vi "Overlay.vi"(0 "Image In":T5, 5 "Overlay Details":T4={"Measurment Name"="", "Measurment Type"="", "Image ID"="", "Result"=[], "PointForOverlays"={"Line"=[], "Angle"=[], "Circle"=[], "Points"={"Points"=[]}, "Coordinate System"={"Origin"={"X"=0.0, "Y"=0.0}, "Angle (deg)"=0.0, "Axis Reference"=0}}, "Color"=16748288, "Mouse coordinates"={"X"=0.0, "Y"=0.0}, "Inspect Overlay Coordinate"=[], "Angle of rotation"=0.0} {"Inspect Overlay Coordinate"."Y" format="%.2f"; "Inspect Overlay Coordinate"."X" format="%.2f"; "Mouse coordinates"."Y" format="%.2f"; "Mouse coordinates"."X" format="%.2f"; "PointForOverlays"."Coordinate System"."Axis Reference" items=["Direct", "Indirect"]; "PointForOverlays"."Coordinate System"."Angle (deg)" format="%.2f"; "PointForOverlays"."Coordinate System"."Origin"."Y" format="%.2f"; "PointForOverlays"."Coordinate System"."Origin"."X" format="%.2f"; "PointForOverlays"."Points"."Points"."Y" format="%.2f"; "PointForOverlays"."Points"."Points"."X" format="%.2f"; "PointForOverlays"."Circle"."Point 2"."Y" format="%.2f"; "PointForOverlays"."Circle"."Point 2"."X" format="%.2f"; "PointForOverlays"."Circle"."Point 1"."Y" format="%.2f"; "PointForOverlays"."Circle"."Point 1"."X" format="%.2f"; "PointForOverlays"."Angle"."line2Point2"."Y" format="%.2f"; "PointForOverlays"."Angle"."line2Point2"."X" format="%.2f"; "PointForOverlays"."Angle"."line2Point1"."Y" format="%.2f"; "PointForOverlays"."Angle"."line2Point1"."X" format="%.2f"; "PointForOverlays"."Angle"."line1Point2"."Y" format="%.2f"; "PointForOverlays"."Angle"."line1Point2"."X" format="%.2f"; "PointForOverlays"."Angle"."line1Point1"."Y" format="%.2f"; "PointForOverlays"."Angle"."line1Point1"."X" format="%.2f"; "PointForOverlays"."Angle"."Point 2a"."Y" format="%.2f"; "PointForOverlays"."Angle"."Point 2a"."X" format="%.2f"; "PointForOverlays"."Angle"."Point 1a"."Y" format="%.2f"; "PointForOverlays"."Angle"."Point 1a"."X" format="%.2f"; "PointForOverlays"."Angle"."vertex"."Y" format="%.2f"; "PointForOverlays"."Angle"."vertex"."X" format="%.2f"; "PointForOverlays"."Angle"."Point 2"."Y" format="%.2f"; "PointForOverlays"."Angle"."Point 2"."X" format="%.2f"; "PointForOverlays"."Angle"."Point 1"."Y" format="%.2f"; "PointForOverlays"."Angle"."Point 1"."X" format="%.2f"; "PointForOverlays"."Line"."Point 2"."Y" format="%.2f"; "PointForOverlays"."Line"."Point 2"."X" format="%.2f"; "PointForOverlays"."Line"."Point 1"."Y" format="%.2f"; "PointForOverlays"."Line"."Point 1"."X" format="%.2f"}, 7 "Testing Parameters":T1={"Stored overlay coordinates"=[], "Testing?"=TRUE}, 9 "Overlay Cluster":T3, 11 "error in":errorcluster) -> (4 "Image Out":T5, 6 "Overlay output":T2, 15 "error out":errorcluster)   [LabVIEW 2015]
uses:
  <vilib>/vision/Image Controls.llb/IMAQ Image.ctl
  Controls/overlayWithDetails.ctl
  Controls/Overlay Cluster.ctl
  Controls/Overlay output.ctl
  Controls/Testing parameters.ctl
  Controls/User inputs (line).ctl
  Controls/Calculated inputs (line).ctl
  Controls/Angle details.ctl
  Controls/Circle dia data.ctl
  Controls/DatumLine draw.ctl
  Controls/GD&T overlay.ctl
panel:
  in  "Xoffset":i32
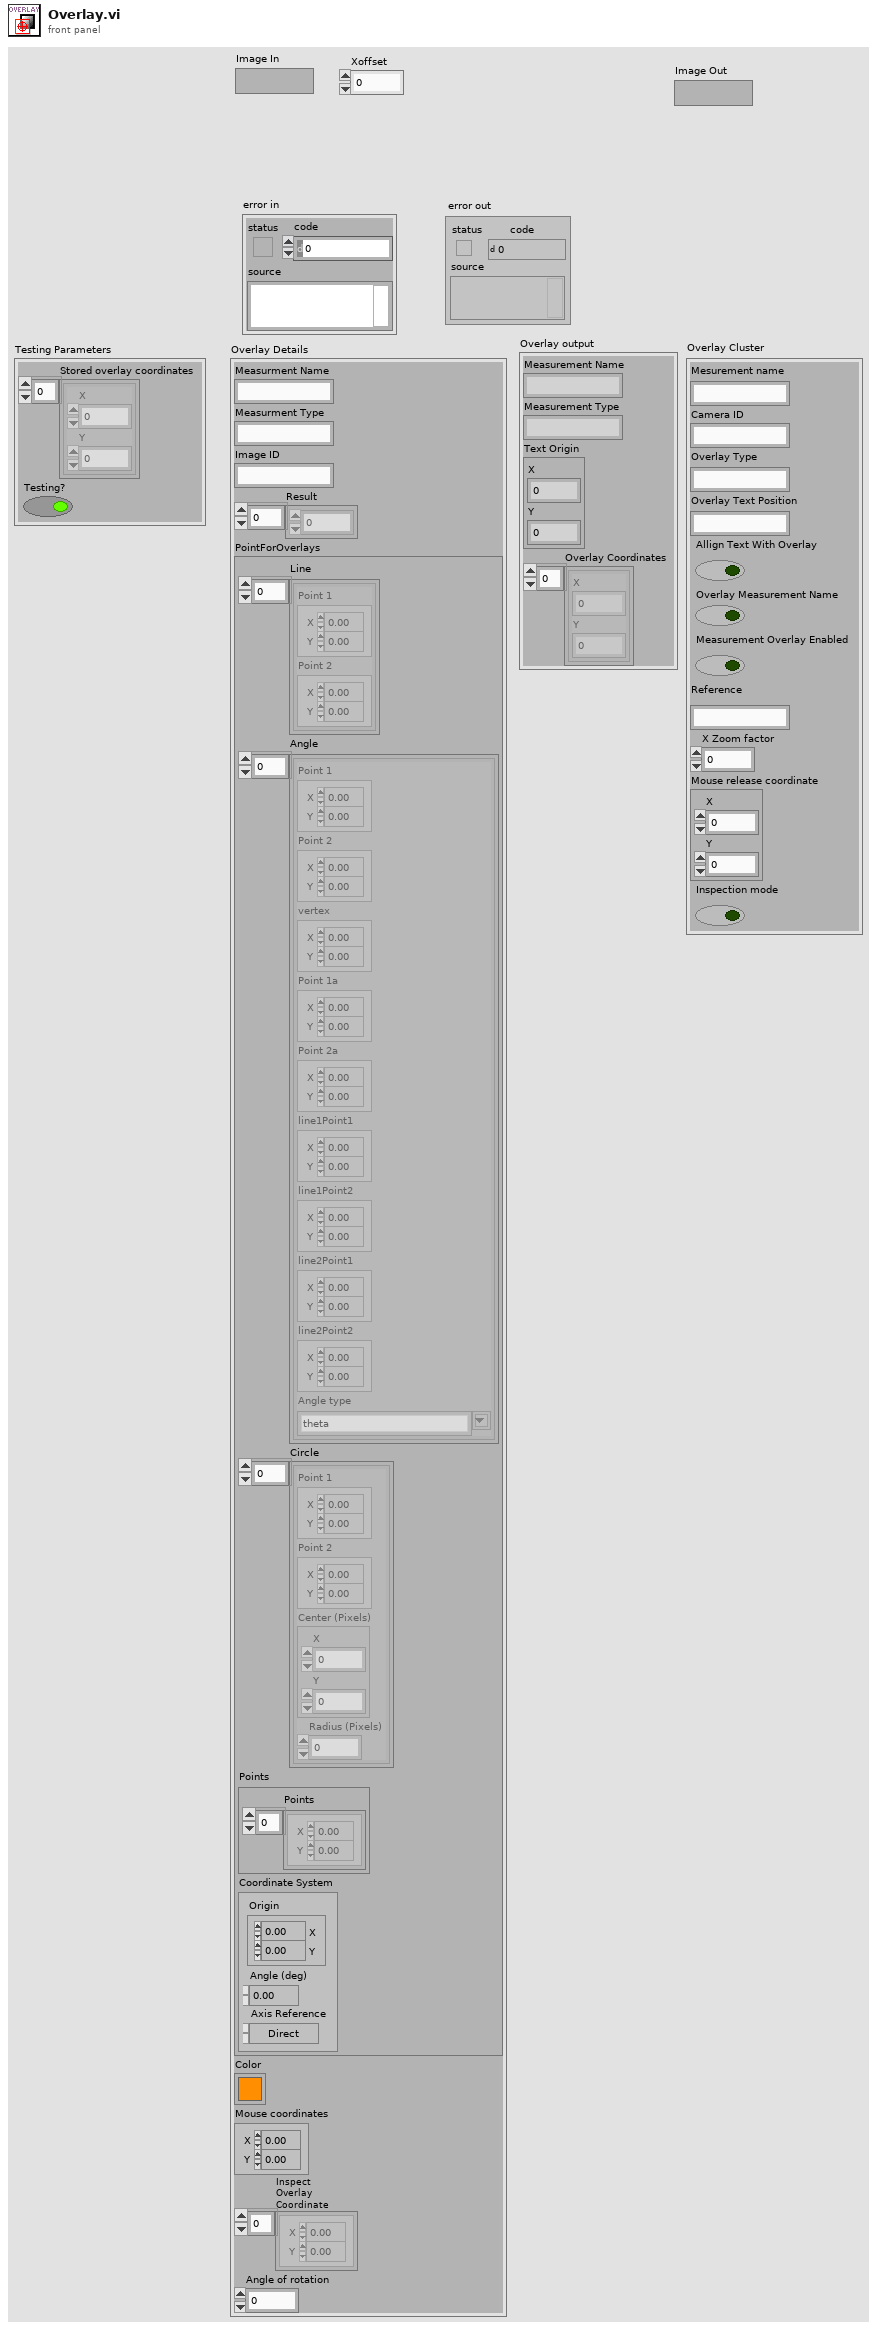
[diagram p1: front panel]
types:
  T1 = typedef "Testing parameters.ctl" = cluster{"Stored overlay coordinates":cluster{"X":sgl, "Y":sgl}[], "Testing?":bool}
  T2 = typedef "Overlay output.ctl" = cluster{"Measurement Name":string, "Measurement Type":string, "Text Origin":cluster{"X":dbl, "Y":dbl}, "Overlay Coordinates":cluster{"X":sgl, "Y":sgl}[]}
  T3 = typedef "Overlay Cluster.ctl" = cluster{"Mesurement name":string, "Camera ID":string, "Overlay Type":string, "Overlay Text Position":string, "Allign Text With Overlay":bool, "Overlay Measurement Name":bool, "Measurement Overlay Enabled":bool, "Reference":string, "X Zoom factor":dbl, "Mouse release coordinate":cluster{"X":dbl, "Y":dbl}, "Inspection mode":bool}
  T4 = typedef "overlayWithDetails.ctl" = cluster{"Measurment Name":string, "Measurment Type":string, "Image ID":string, "Result":sgl[], "PointForOverlays":cluster{"Line":cluster{"Point 1":cluster{"X":sgl, "Y":sgl}, "Point 2":cluster{"X":sgl, "Y":sgl}}[], "Angle":cluster{"Point 1":cluster{"X":sgl, "Y":sgl}, "Point 2":cluster{"X":sgl, "Y":sgl}, "vertex":cluster{"X":sgl, "Y":sgl}, "Point 1a":cluster{"X":sgl, "Y":sgl}, "Point 2a":cluster{"X":sgl, "Y":sgl}, "line1Point1":cluster{"X":sgl, "Y":sgl}, "line1Point2":cluster{"X":sgl, "Y":sgl}, "line2Point1":cluster{"X":sgl, "Y":sgl}, "line2Point2":cluster{"X":sgl, "Y":sgl}, "Angle type":string}[], "Circle":cluster{"Point 1":cluster{"X":sgl, "Y":sgl}, "Point 2":cluster{"X":sgl, "Y":sgl}, "Center (Pixels)":cluster{"X":sgl, "Y":sgl}, "Radius (Pixels)":dbl}[], "Points":cluster{"Points":cluster{"X":sgl, "Y":sgl}[]}, "Coordinate System":cluster{"Origin":cluster{"X":sgl, "Y":sgl}, "Angle (deg)":sgl, "Axis Reference":u32}}, "Color":u32, "Mouse coordinates":cluster{"X":sgl, "Y":sgl}, "Inspect Overlay Coordinate":cluster{"X":sgl, "Y":sgl}[], "Angle of rotation":dbl}
  T5 = typedef "IMAQ Image.ctl" = refnum<image>
  T6 = cluster{"Inspection mode":bool, "Overlay coordinates":cluster{"X":sgl, "Y":sgl}[], "Config coordinates":cluster{"X":sgl, "Y":sgl}[]}
  T7 = typedef "Angle details.ctl" = cluster{"Text factor":u8, "Xoffset":i32, "Arc size":dbl, "Result":sgl, "Line width":i32, "Measurment Name":string, "Angle":cluster{"Point 1":cluster{"X":sgl, "Y":sgl}, "Point 2":cluster{"X":sgl, "Y":sgl}, "vertex":cluster{"X":sgl, "Y":sgl}, "Point 1a":cluster{"X":sgl, "Y":sgl}, "Point 2a":cluster{"X":sgl, "Y":sgl}, "line1Point1":cluster{"X":sgl, "Y":sgl}, "line1Point2":cluster{"X":sgl, "Y":sgl}, "line2Point1":cluster{"X":sgl, "Y":sgl}, "line2Point2":cluster{"X":sgl, "Y":sgl}, "Angle type":string}, "Maintain Width?":bool, "Size factor":u32, "Colour":u32, "Mouse release point":cluster{"X":sgl, "Y":sgl}, "Small FOV?":bool, "Fixed FOV parameters":cluster{"Inspection mode":bool, "Overlay coordinates":cluster{"X":sgl, "Y":sgl}[], "Config coordinates":cluster{"X":sgl, "Y":sgl}[]}}
  T8 = typedef "Circle dia data.ctl" = cluster{"Overlay shift":dbl, "Xoffset":i32, "Arc size":dbl, "Measurement type":string, "Result":sgl, "Text size factor":u32, "Measurment Name":string, "Colour":u32, "Pixel density":dbl, "Circle":cluster{"Point 1":cluster{"X":sgl, "Y":sgl}, "Point 2":cluster{"X":sgl, "Y":sgl}, "Center (Pixels)":cluster{"X":sgl, "Y":sgl}, "Radius (Pixels)":dbl}, "Line width":i32, "Input points":cluster{"slanting line start poing":cluster{"X":sgl, "Y":sgl}, "Sleeping line start point":cluster{"X":sgl, "Y":sgl}}, "Mouse coordinates":cluster{"X":sgl, "Y":sgl}, "Size factor":sgl, "Inspect Overlay Coordinates":cluster{"X":sgl, "Y":sgl}[], "Config Overlay Coordinates":cluster{"X":sgl, "Y":sgl}[]}
  T9 = cluster{"slanting line start poing":cluster{"X":sgl, "Y":sgl}, "Sleeping line start point":cluster{"X":sgl, "Y":sgl}}
  T10 = cluster{"Overlay coordinates":cluster{"X":dbl, "Y":dbl}[], "Config coordinates":cluster{"X":dbl, "Y":dbl}[], "Inspection mode?":bool}
  T11 = typedef "DatumLine draw.ctl" = cluster{"Angle":dbl, "Reference":string, "Xoffset":i32, "Arc size":dbl, "Measurment Name":string, "Pixel density":dbl, "Circle":cluster{"Point 1":cluster{"X":sgl, "Y":sgl}, "Point 2":cluster{"X":sgl, "Y":sgl}, "Center (Pixels)":cluster{"X":sgl, "Y":sgl}, "Radius (Pixels)":dbl}, "Color":u32, "Slanting line start":cluster{"X":sgl, "Y":sgl}, "Sleeping line start":cluster{"X":sgl, "Y":sgl}, "Mouse release":cluster{"X":sgl, "Y":sgl}, "Line width":i32, "Small FOV?":bool, "Fixed overlay details":cluster{"Overlay coordinates":cluster{"X":dbl, "Y":dbl}[], "Config coordinates":cluster{"X":dbl, "Y":dbl}[], "Inspection mode?":bool}, "PM angle":dbl}
  T12 = cluster{"Point 1":cluster{"X":sgl, "Y":sgl}, "Point 2":cluster{"X":sgl, "Y":sgl}, "Center (Pixels)":cluster{"X":sgl, "Y":sgl}, "Radius (Pixels)":dbl}
  T13 = typedef "GD&T overlay.ctl" = cluster{"Overlay shift":dbl, "Reference":string, "Arc size":dbl, "Measurement type":string, "Xoffset":i32, "Result":sgl, "Measurment Name":string, "Color":u32, "Points":cluster{"Point 1":cluster{"X":sgl, "Y":sgl}, "Point 2":cluster{"X":sgl, "Y":sgl}, "Center (Pixels)":cluster{"X":sgl, "Y":sgl}, "Radius (Pixels)":dbl}, "Pixel density":dbl, "Line width":i32, "Mouse release point":cluster{"X":dbl, "Y":dbl}, "Slanting start point":cluster{"X":dbl, "Y":dbl}, "Sleeping start point":cluster{"X":dbl, "Y":dbl}, "Small FOV?":bool, "Fixed overlays":cluster{"Overlay coordinates":cluster{"X":dbl, "Y":dbl}[], "Config coordinates":cluster{"X":dbl, "Y":dbl}[], "Inspection mode":bool}, "Angle of rotation":dbl}
  T14 = cluster{"Arrow height":dbl, "Measurment Name":string, "Coordinate System":cluster{"Origin":cluster{"X":sgl, "Y":sgl}, "Angle (deg)":sgl, "Axis Reference":u32}, "Color":u32, "Width":u32, "Arrow angle in":dbl, "SmallFOV?":bool}
  T15 = cluster{"Xoffset":i32, "Point size":dbl, "Arc size":dbl, "Measurment Name":string, "Circle":cluster{"Point 1":cluster{"X":sgl, "Y":sgl}, "Point 2":cluster{"X":sgl, "Y":sgl}, "Center (Pixels)":cluster{"X":sgl, "Y":sgl}, "Radius (Pixels)":dbl}, "Color":u32, "Line width":i32}
  T16 = cluster{"Line":cluster{"Point 1":cluster{"X":sgl, "Y":sgl}, "Point 2":cluster{"X":sgl, "Y":sgl}}[], "Angle":cluster{"Point 1":cluster{"X":sgl, "Y":sgl}, "Point 2":cluster{"X":sgl, "Y":sgl}, "vertex":cluster{"X":sgl, "Y":sgl}, "Point 1a":cluster{"X":sgl, "Y":sgl}, "Point 2a":cluster{"X":sgl, "Y":sgl}, "line1Point1":cluster{"X":sgl, "Y":sgl}, "line1Point2":cluster{"X":sgl, "Y":sgl}, "line2Point1":cluster{"X":sgl, "Y":sgl}, "line2Point2":cluster{"X":sgl, "Y":sgl}, "Angle type":string}[], "Circle":cluster{"Point 1":cluster{"X":sgl, "Y":sgl}, "Point 2":cluster{"X":sgl, "Y":sgl}, "Center (Pixels)":cluster{"X":sgl, "Y":sgl}, "Radius (Pixels)":dbl}[], "Points":cluster{"Points":cluster{"X":sgl, "Y":sgl}[]}, "Coordinate System":cluster{"Origin":cluster{"X":sgl, "Y":sgl}, "Angle (deg)":sgl, "Axis Reference":u32}}
  T17 = cluster{"Arrow height":dbl, "Point size":dbl, "Arc size":dbl}
  T18 = cluster{"Point 1":cluster{"X":sgl, "Y":sgl}, "Point 2":cluster{"X":sgl, "Y":sgl}, "vertex":cluster{"X":sgl, "Y":sgl}, "Point 1a":cluster{"X":sgl, "Y":sgl}, "Point 2a":cluster{"X":sgl, "Y":sgl}, "line1Point1":cluster{"X":sgl, "Y":sgl}, "line1Point2":cluster{"X":sgl, "Y":sgl}, "line2Point1":cluster{"X":sgl, "Y":sgl}, "line2Point2":cluster{"X":sgl, "Y":sgl}, "Angle type":string}[]
  T19 = cluster{"Point 1":cluster{"X":sgl, "Y":sgl}, "Point 2":cluster{"X":sgl, "Y":sgl}, "Center (Pixels)":cluster{"X":sgl, "Y":sgl}, "Radius (Pixels)":dbl}[]
  T20 = cluster{"Point 1":cluster{"X":sgl, "Y":sgl}, "Point 2":cluster{"X":sgl, "Y":sgl}}[]
  T21 = typedef "Calculated inputs (line).ctl" = cluster{"Arrow head diverge angle":dbl, "Arrow height":dbl, "Line width":i32, "Maintain Width?":bool, "Text factor":u8}
  T22 = typedef "User inputs (line).ctl" = cluster{"Measurement name":string, "Line":cluster{"Point 1":cluster{"X":sgl, "Y":sgl}, "Point 2":cluster{"X":sgl, "Y":sgl}}, "Result":sgl, "Overlay shift1":dbl, "Overlay shift2":dbl, "Allign Text With Overlay":bool, "Overlay text position":string, "Color":u32, "Xoffset":i32, "Size factor":dbl, "Inspection mode?":bool, "Configuration overlay coordinates":cluster{"X":sgl, "Y":sgl}[]}
  T23 = cluster{"Point 1":cluster{"X":sgl, "Y":sgl}, "Point 2":cluster{"X":sgl, "Y":sgl}}
  T24 = cluster{"Origin":cluster{"X":sgl, "Y":sgl}, "Angle (deg)":sgl, "Axis Reference":u32}
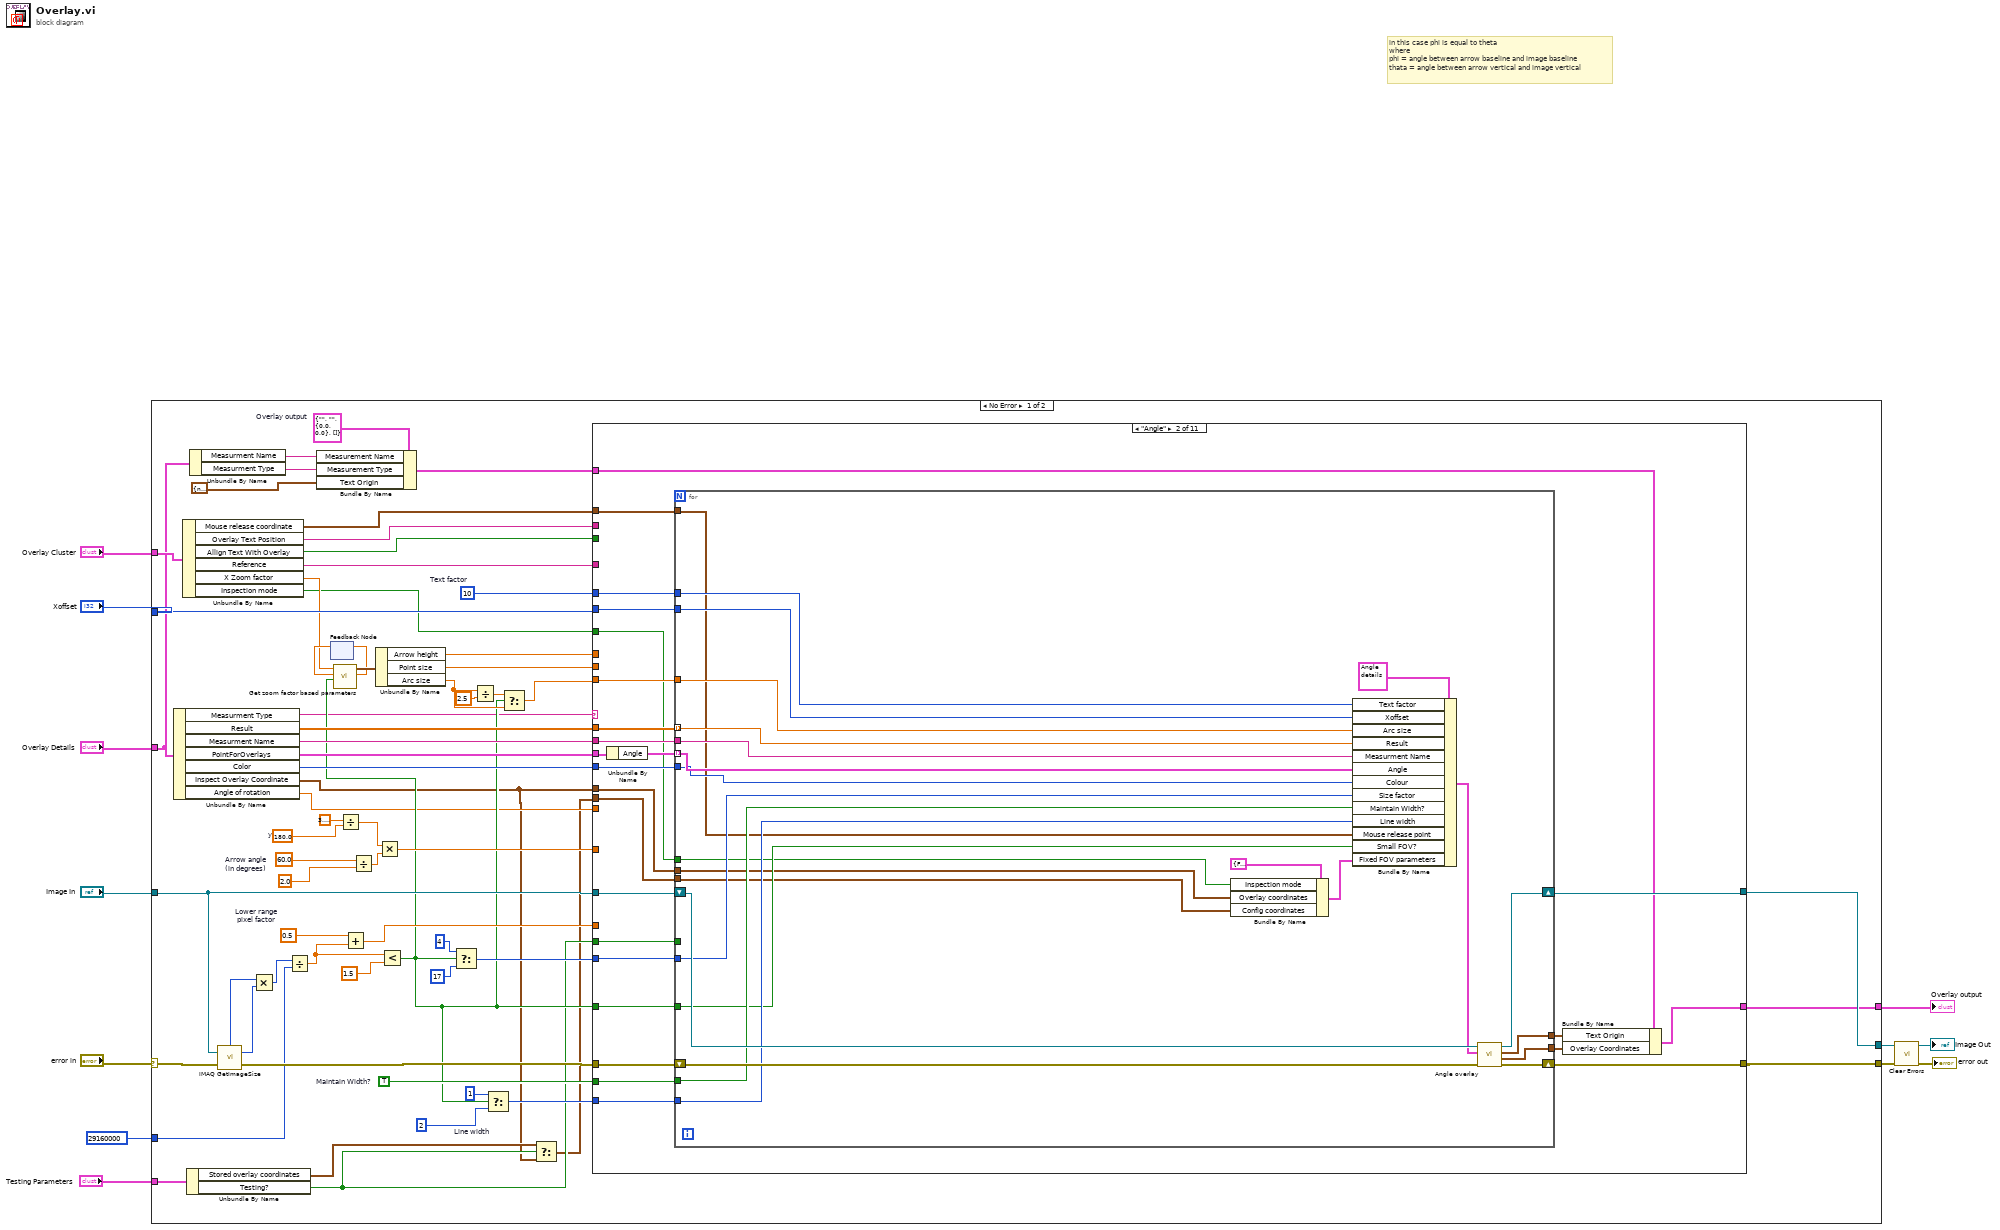
[diagram p0: block diagram]
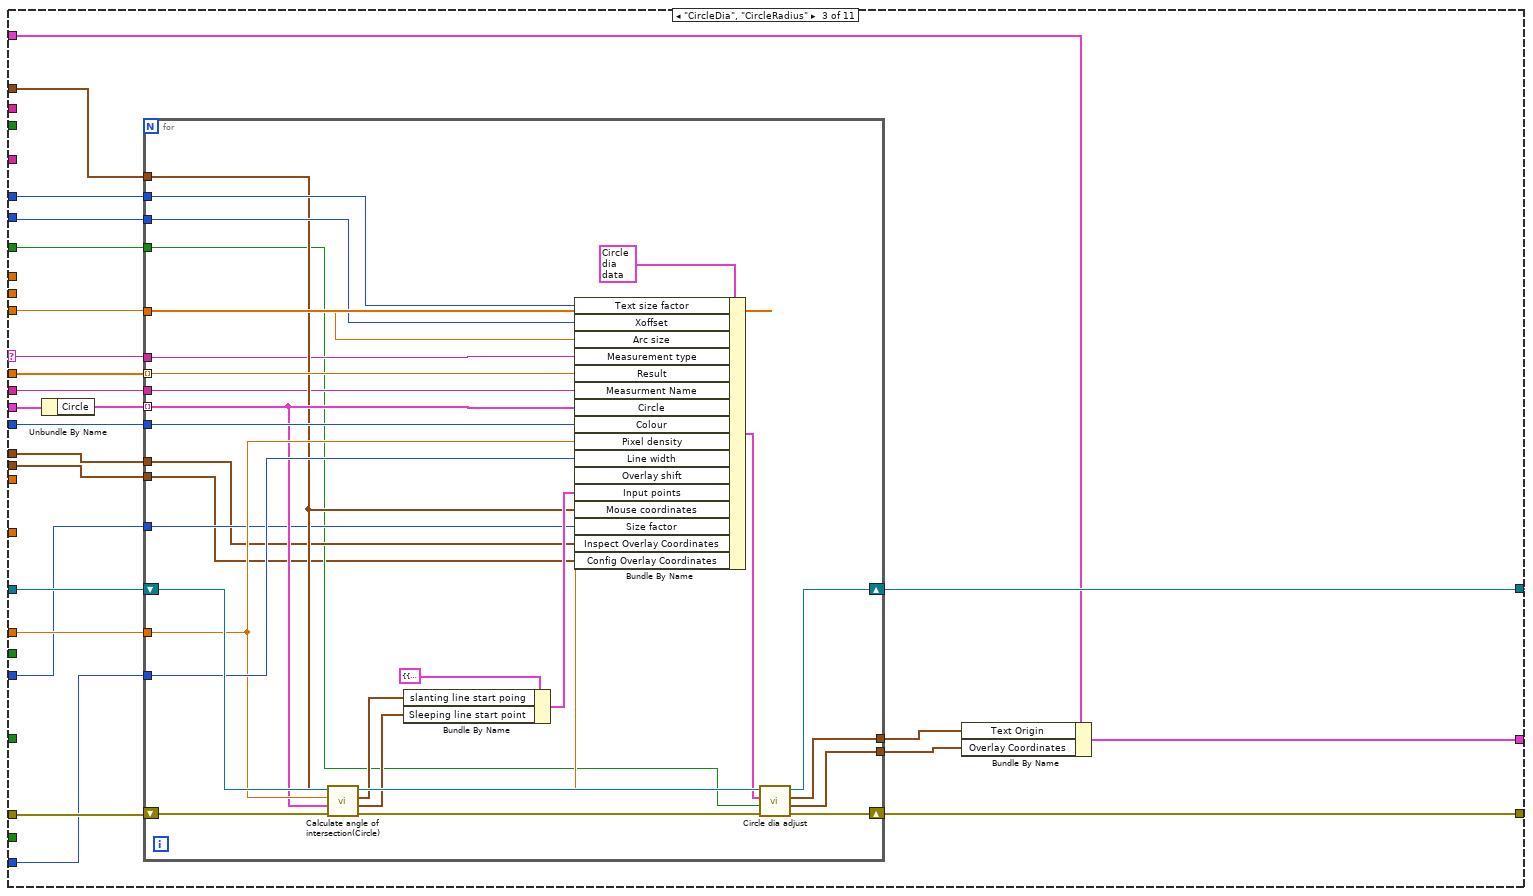
[diagram p3: hidden frame]
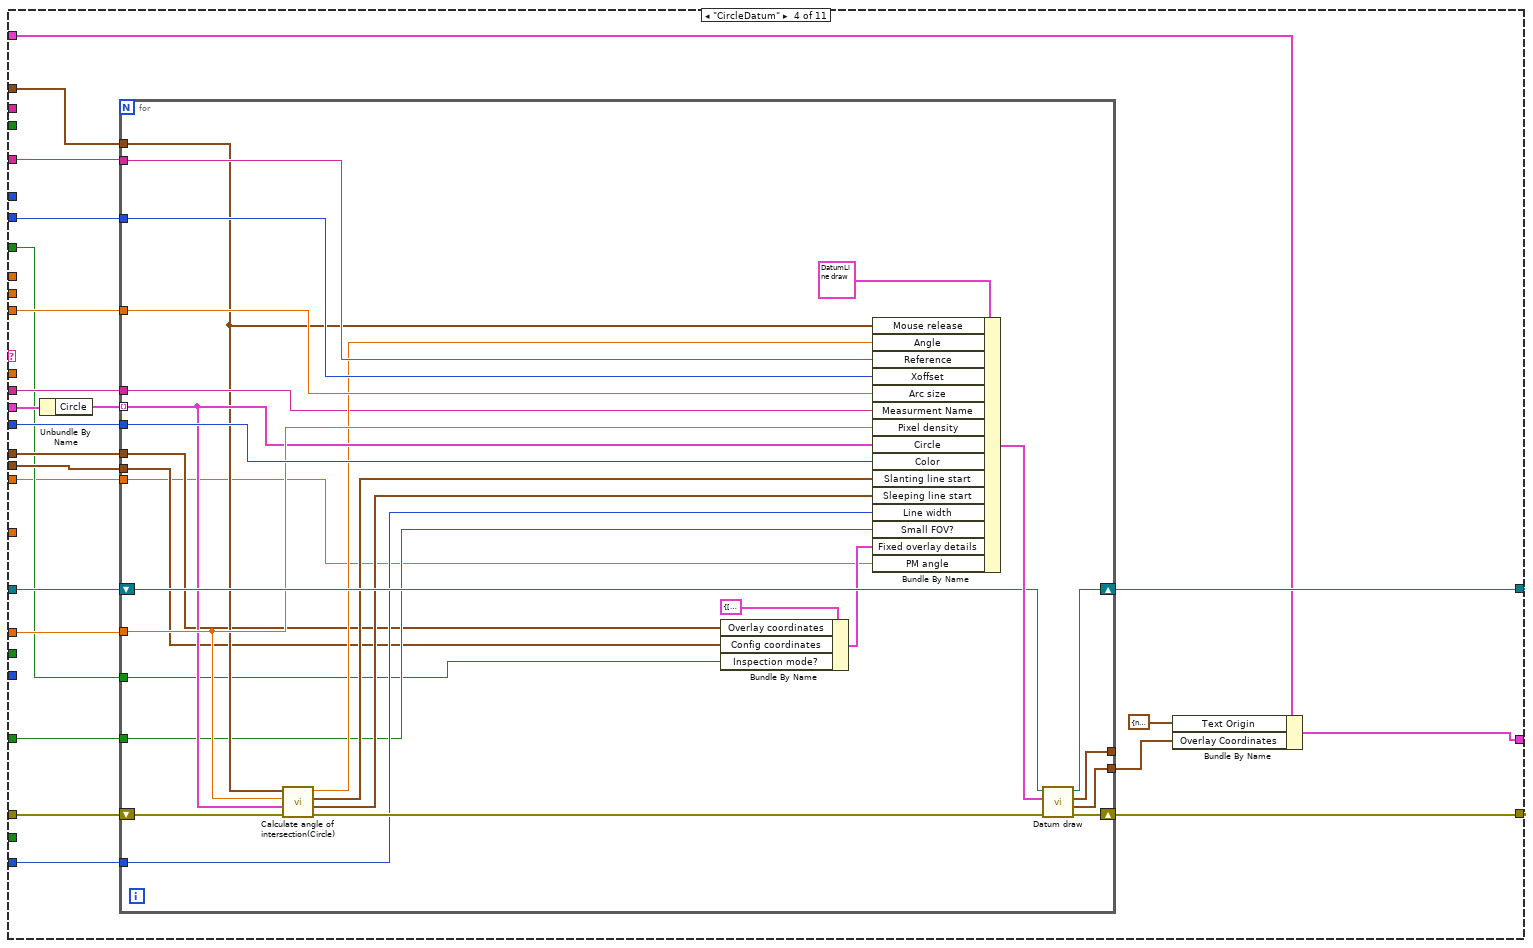
[diagram p4: hidden frame]
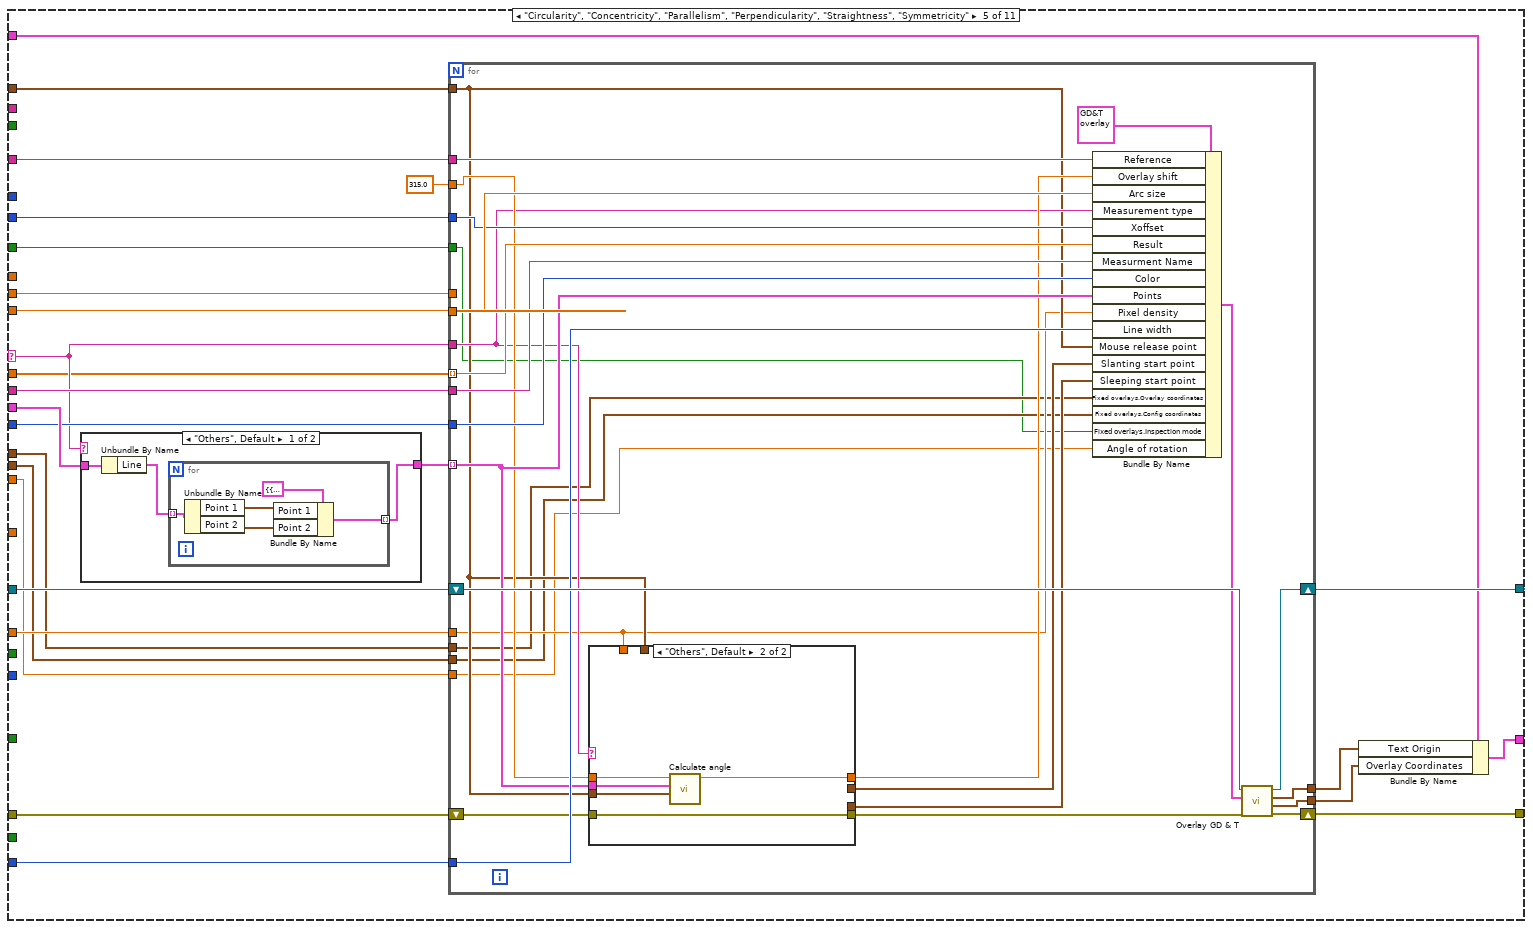
[diagram p5: hidden frame]
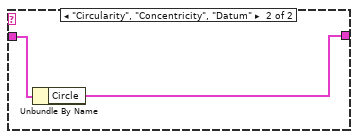
[diagram p6: hidden frame]
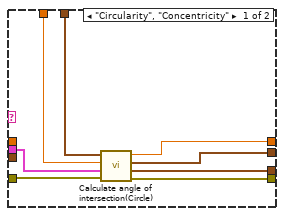
[diagram p7: hidden frame]
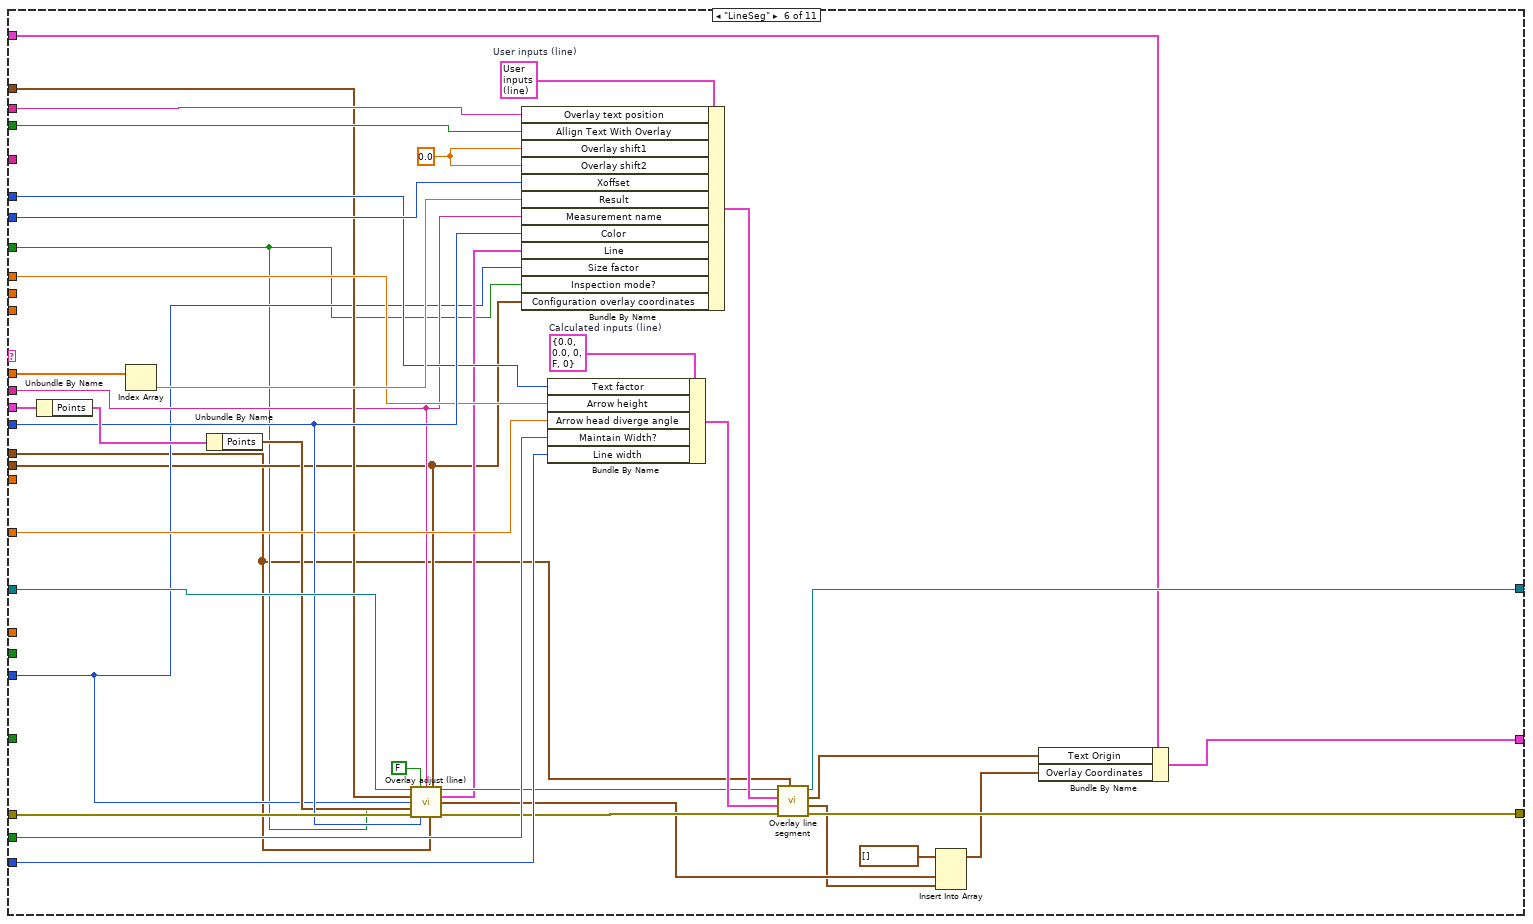
[diagram p8: hidden frame]
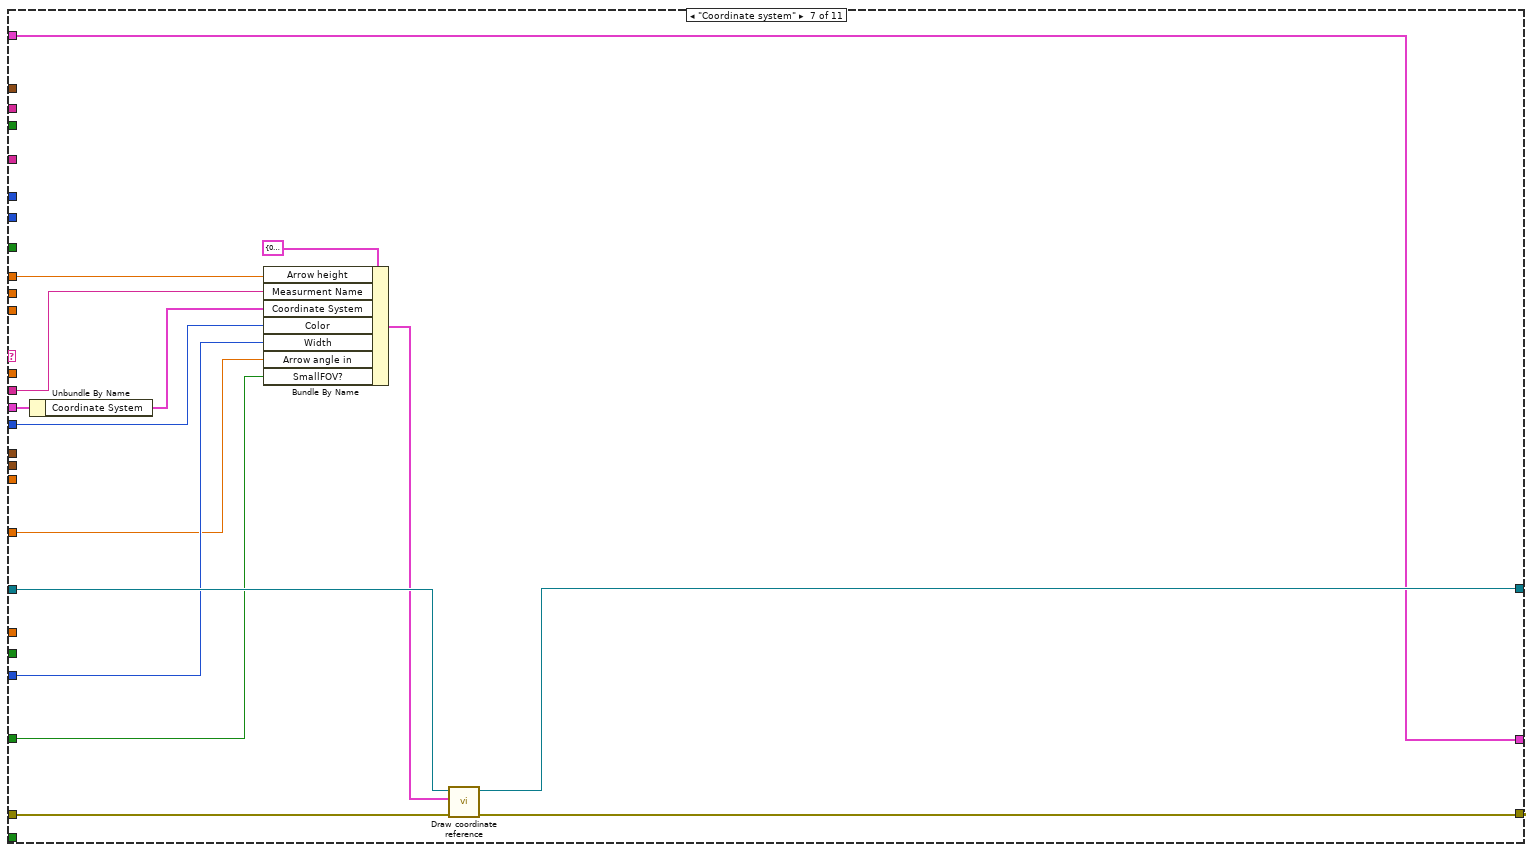
[diagram p9: hidden frame]
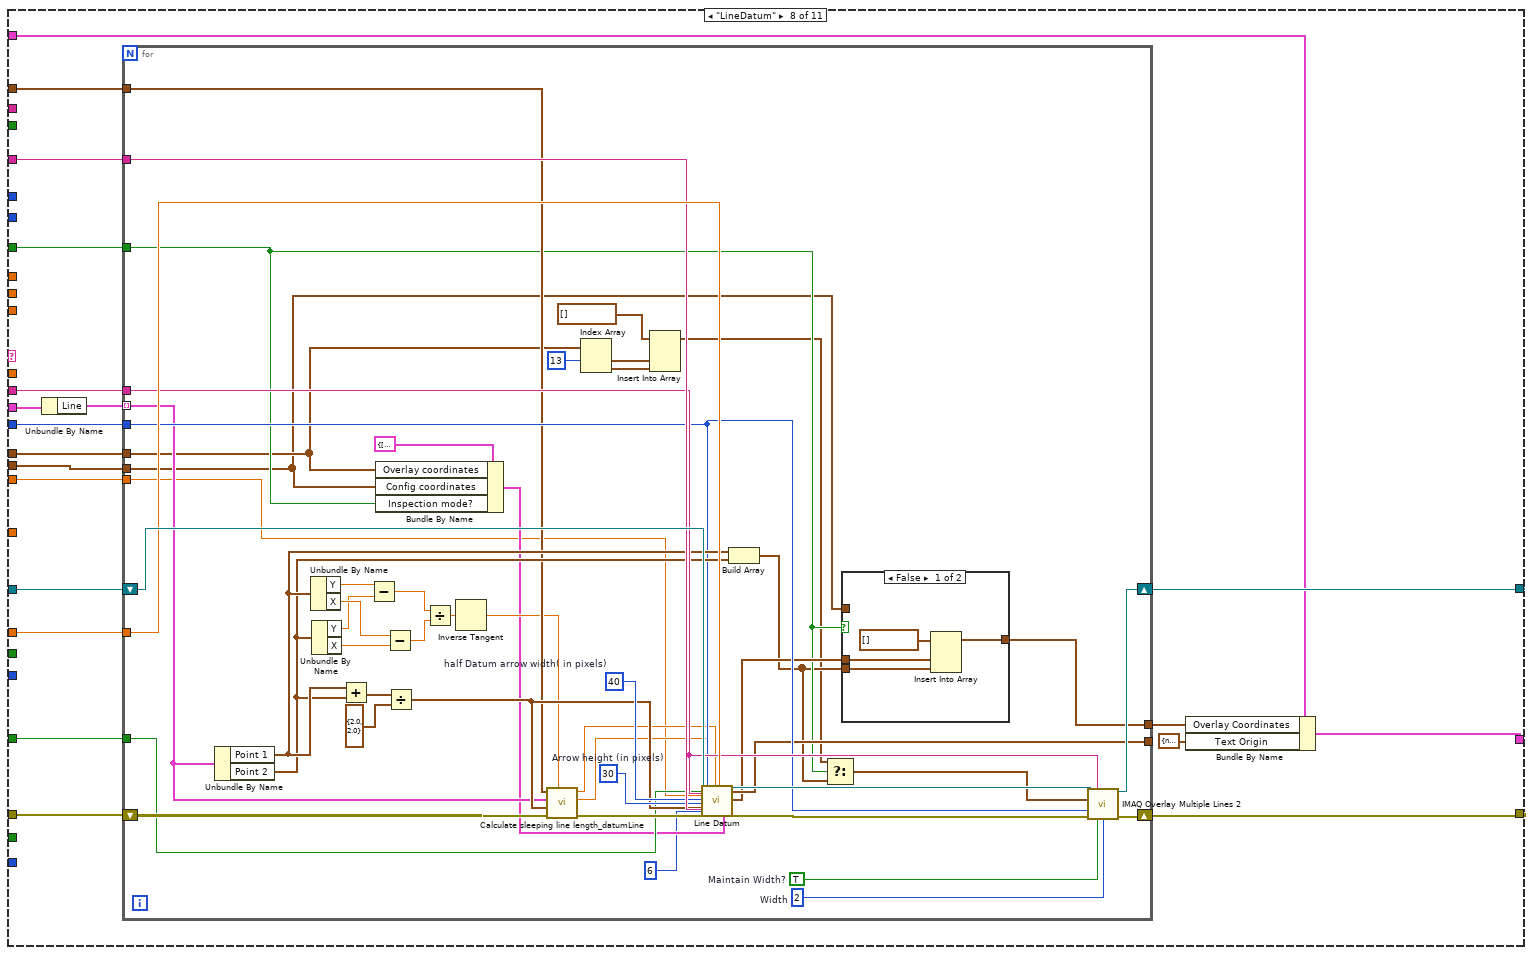
[diagram p10: hidden frame]
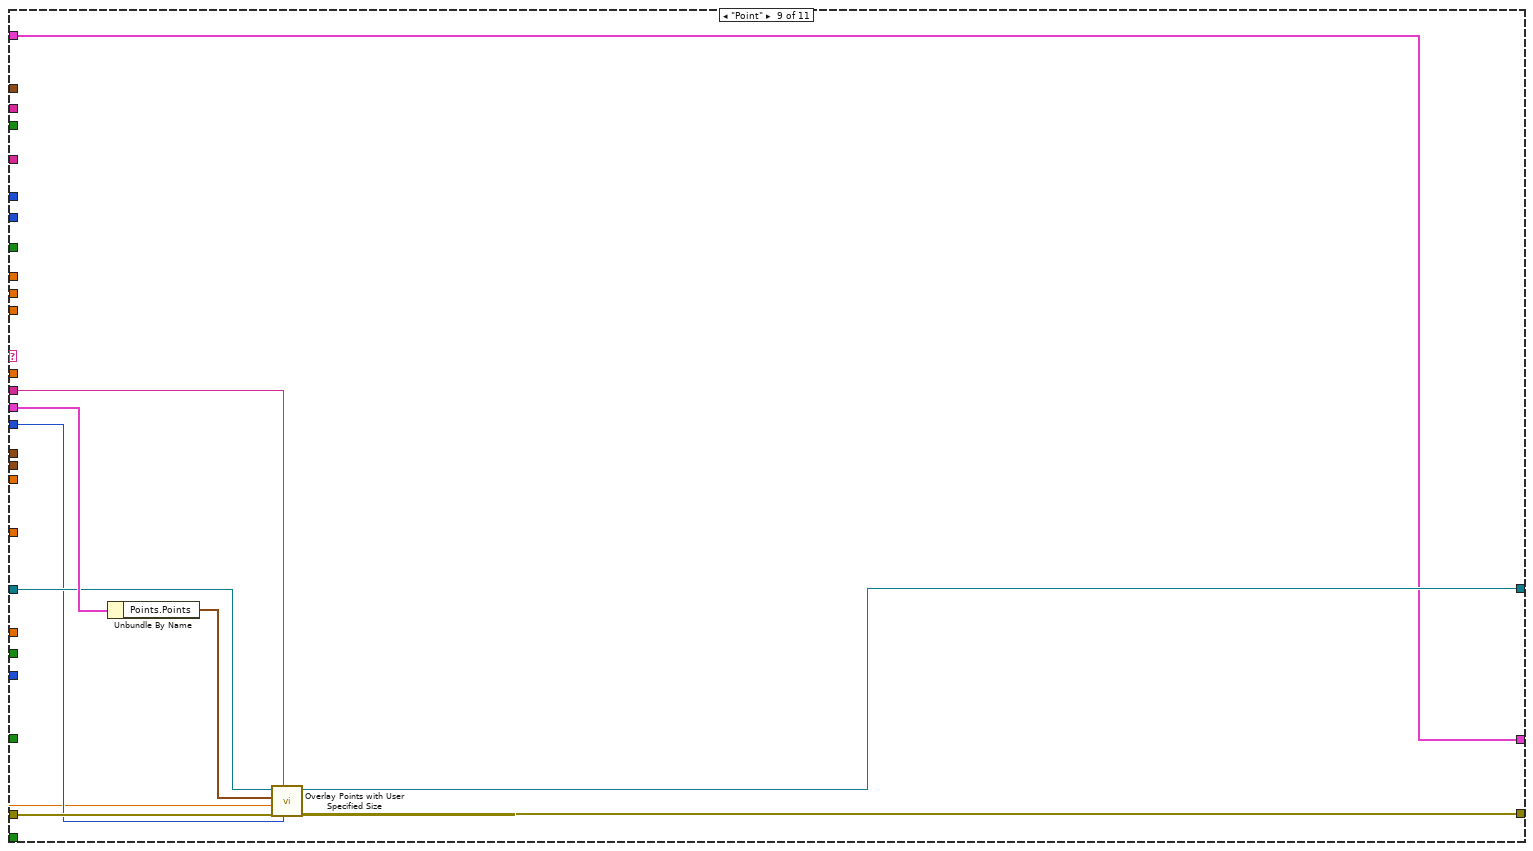
[diagram p12: hidden frame]
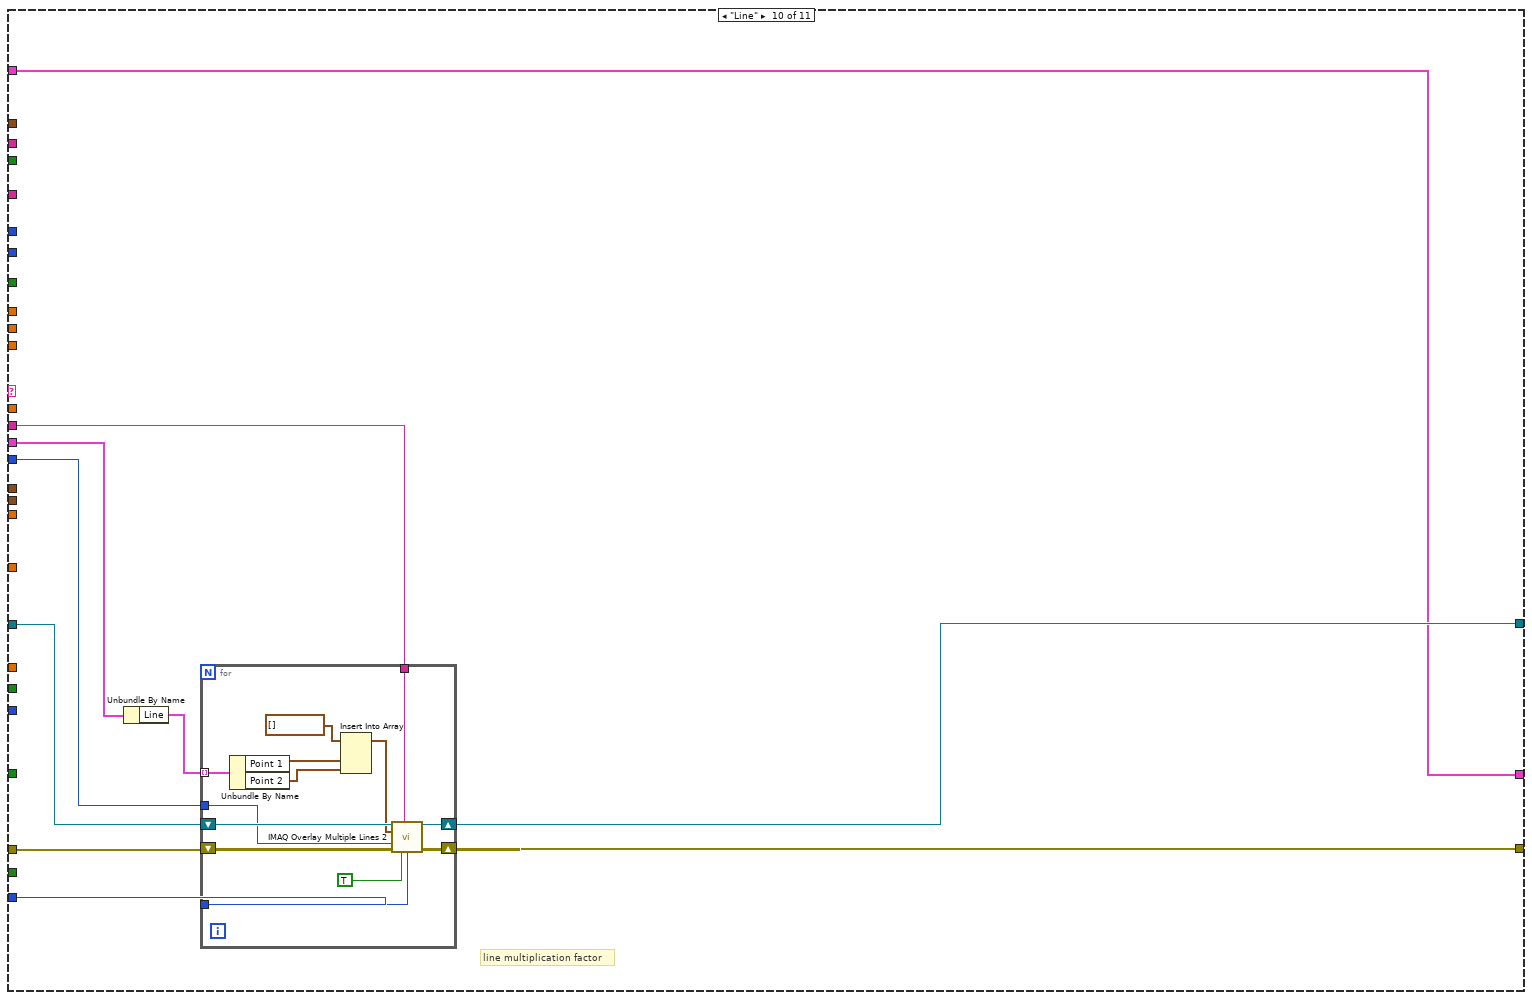
[diagram p13: hidden frame]
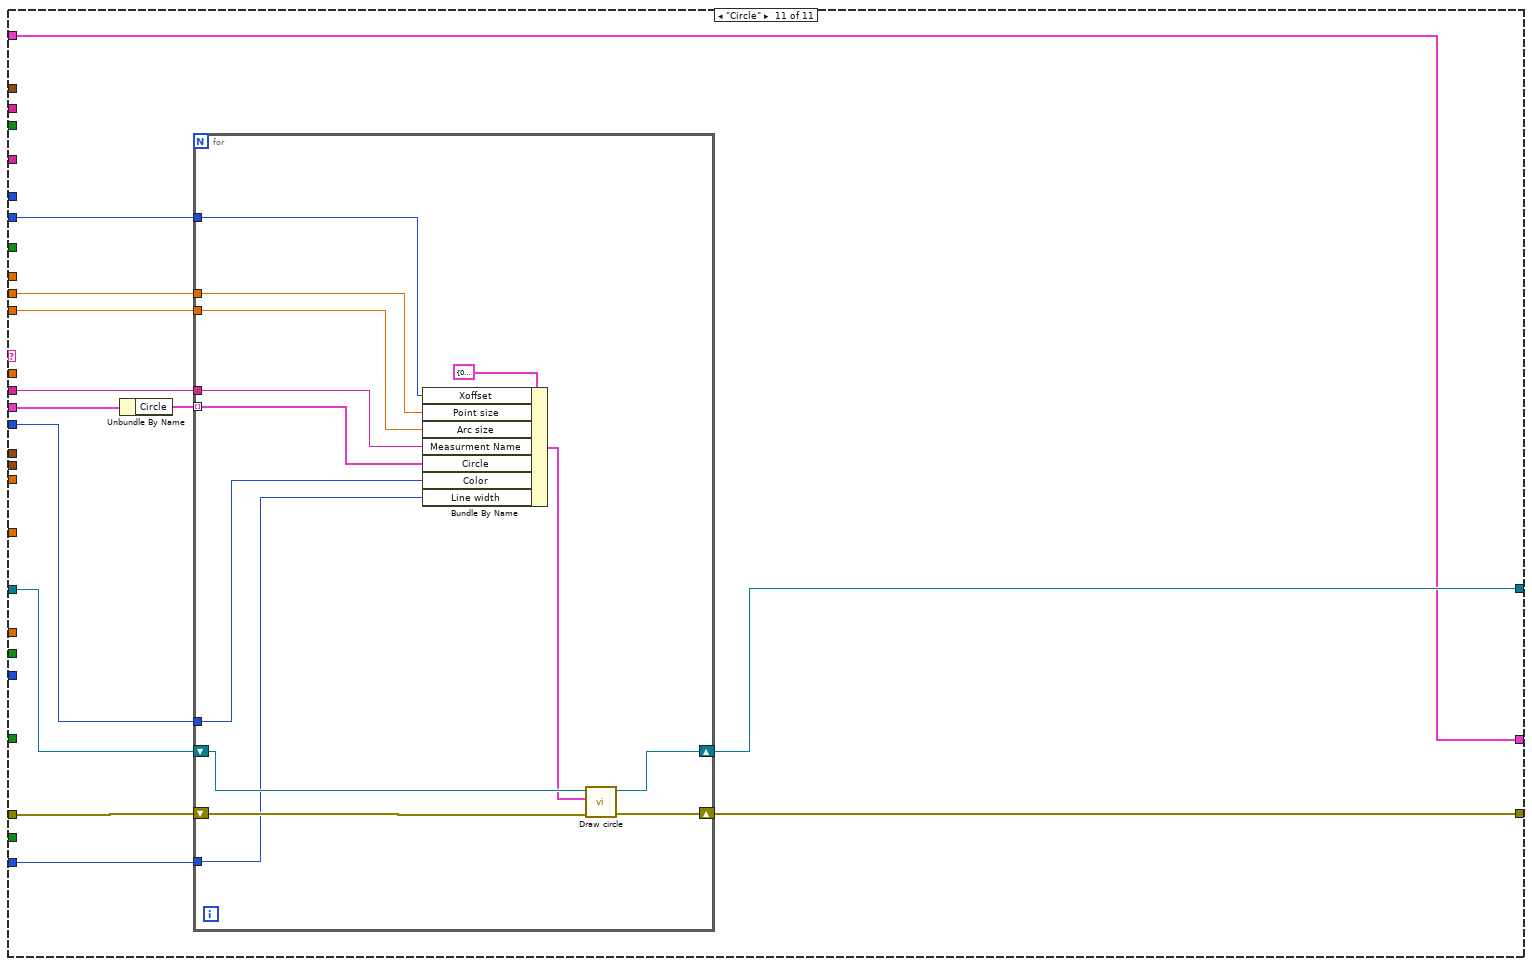
[diagram p14: hidden frame]
diagram:
  # "in this case phi is equal to theta\nwhere\nphi = angle between arrow baseline and image baseline\nthata = angle between arrow vertical and image vertical"
  n1 = case shown="No Error" "error in" {
    selector: "error in" -> [w69 w500]
    tunnel: "Image In" -> [w67 w499]
    tunnel: [w75 w499] -> w10
    tunnel: [w74 w500] -> w5
    tunnel: "Xoffset" -> [w73 _]
    tunnel: "Overlay Details" -> [w33 _]
    tunnel: "Overlay Cluster" -> [w61 _]
    tunnel: u64 29160000 ("y") -> [w58 _]
    tunnel: [w34 _] -> w2
    tunnel: "Testing Parameters" -> [w16 _]
    frame No Error {
      w20 = T2 {"Measurement Name"="", "Measurement Type"="", "Text Origin"={"X"=0.0, "Y"=0.0}, "Overlay Coordinates"=[]}  # Overlay output
      w38 = 0.5  # Lower range  pixel factor
      w50 = 60.0  # Arrow angle  (in degrees)
      w52 = 180.0  # y
      w28 = 2  # Line width
      w54 = TRUE  # Maintain Width?
      w62 = u8 10  # Text factor
      n2 = Unbundle By Name(w33) -> ("Measurment Type"=w17:string, "Result"=w72:sgl[], "Measurment Name"=w63:string, "PointForOverlays"=w71:T16, "Color"=w70:u32, "Inspect Overlay Coordinate"=w13:cluster{"X":sgl, "Y":sgl}[], "Angle of rotation"=w18:dbl)
      n3 = Unbundle By Name(w61) -> ("Mouse release coordinate"=w35:cluster{"X":dbl, "Y":dbl}, "Overlay Text Position"=w36:string, "Allign Text With Overlay"=w37:bool, "Reference"=w60:string, "X Zoom factor"=w40:dbl, "Inspection mode"=w19:bool)
      n4 = Unbundle By Name(w16) -> ("Stored overlay coordinates"=w14:cluster{"X":sgl, "Y":sgl}[], "Testing?"=w15:bool)
      n5 = Unbundle By Name(w33) -> ("Measurment Name"=w32:string, "Measurment Type"=w31:string)
      n6 = call "IMAQ GetImageSize"("Image"=w67, "error in (no error)"=w69) -> ("Y Resolution"=w66:i32, "X Resolution"=w65:i32, "error out"=w68:errorcluster)  [unwired: 2 in]
      n7 = Multiply(x=w65, y=w66) -> (x*y=w59:i32)
      n8 = Divide(x=w59, y=w58) -> (x/y=w39:dbl)
      n9 = Bundle By Name(cluster=w20, "Measurement Name"=w32, "Measurement Type"=w31, "Text Origin"=cluster{"X":dbl, "Y":dbl} {"X"=nan, "Y"=nan}) -> (w29:T2)
      n10 = feedback #1() -> (w41:dbl)  [unwired: 1 in]
      n11 = Divide(x=3.141592653589793, y=w52) -> (x/y=w51:dbl)
      n12 = Add(x=w38, y=w39) -> (x+y=w64:dbl)
      n13 = Divide(x=w50, y=2.0) -> (x/y=w49:dbl)
      n14 = Multiply(x=w51, y=w49) -> (x*y=w47:dbl)
      n15 = Less?(x=w39, y=1.5) -> (x < y?=w21:bool)
      n16 = call "Get zoom factor based parameters.vi"("Small FOV?"=w21, "Zoom factor\nprevious iteration\nvalue in"=w41, "Zoom factor\ncompare"=w40) -> ("Zoom factor\nprevious iteration\nvalue"=w46:dbl, "Overlay variations"=w57:T17)  [unwired: 6 in, 1 out]
      n17 = feedback-in #1(w46) -> ()
      n18 = Unbundle By Name(w57) -> ("Arrow height"=w56:dbl, "Point size"=w55:dbl, "Arc size"=w23:dbl)
      n19 = Select(t=u32 4 ("Color"), s=w21, f=u32 17 ("Color")) -> (s? t:f=w42:u32)
      n20 = Divide(x=w23, y=2.5) -> (x/y=w25:dbl)
      n21 = Select(t=1, s=w21, f=w28) -> (s? t:f=w26:i32)
      n22 = Select(t=w25, s=w21, f=w23) -> (s? t:f=w22:dbl)
      n23 = Select(t=w14, s=w15, f=w13) -> (s? t:f=w12:cluster{"X":sgl, "Y":sgl}[])
      n24 = case shown="\"Angle\"" w17 {
        selector: w17 -> [_ _ w140 _ w252 _ _ _ _ _ _]
        tunnel: w67 -> [w77 w99 w144 w197 w249 w349 w362 w381 w446 w458 w477]
        tunnel: [w77 w103 w151 w203 w257 w348 w364 w380 w444 w457 w478] -> w75
        tunnel: [w78 w102 w152 w204 w258 w347 w363 w378 w445 w456 w482] -> w74
        tunnel: w63 -> [_ w94 w145 w199 w253 w331 w360 w375 w442 w453 w476]
        tunnel: w72 -> [_ w101 w150 _ w247 w341 _ _ _ _ _]
        tunnel: w68 -> [w78 w100 w143 w195 w248 w346 w353 w379 w448 w459 w483]
        tunnel: w71 -> [_ w97 w148 w201 w255 w344 w359 w384 w449 w455 w485]
        tunnel: w73 -> [_ w98 w149 w202 w256 w345 _ _ _ _ w481]
        tunnel: w70 -> [_ w95 w146 w200 w254 w342 w357 w382 w443 w452 w479]
        tunnel: w60 -> [_ _ _ w198 w250 _ _ w377 _ _ _]
        tunnel: w64 -> [_ _ w142 w194 w246 _ _ w376 _ _ _]
        tunnel: w26 -> [_ w90 w134 w188 w243 w333 _ _ _ w451 w480]
        tunnel: w62 -> [_ w93 w141 _ _ w339 _ _ _ _ _]
        tunnel: w56 -> [_ _ _ _ _ w337 w361 _ _ _ _]
        tunnel: w55 -> [_ _ _ _ w244 _ _ _ w441 _ w475]
        tunnel: w22 -> [_ w91 w139 w193 w245 _ _ _ _ _ w474]
        tunnel: w54 -> [_ w92 _ _ _ w334 _ _ _ _ _]
        tunnel: w47 -> [_ _ _ _ _ w338 w355 _ _ _ _]
        tunnel: w42 -> [_ w89 w133 _ _ w318 w356 _ _ _ _]
        tunnel: w37 -> [_ _ _ _ _ w335 _ _ _ _ _]
        tunnel: w36 -> [_ _ _ _ _ w336 _ _ _ _ _]
        tunnel: w35 -> [_ w88 w138 w192 w241 w332 _ w374 _ _ _]
        tunnel: [w76 w85 w136 w190 w238 w330 w352 w372 w440 w450 w473] -> w34
        tunnel: w29 -> [w76 w87 w135 w191 w240 w329 w352 w373 w440 w450 w473]
        tunnel: w21 -> [_ w84 _ w187 _ _ w350 w370 _ _ _]
        tunnel: w13 -> [_ w82 w131 w186 w236 w314 _ w369 _ _ _]
        tunnel: w19 -> [_ w83 w130 w184 w234 w315 _ w367 _ _ _]
        tunnel: w12 -> [_ w81 w129 w185 w235 w316 _ w368 _ _ _]
        tunnel: w18 -> [_ _ _ w182 w233 _ _ w365 _ _ _]
        tunnel: w15 -> [_ w79 _ _ _ _ _ _ _ _ _]
        frame Default {
        }
        frame "Angle" {
          n25 = Unbundle By Name(w97) -> ("Angle"=w96:T18)
          n26 = for {
            tunnel: w101 -> [w120] mode=indexing
            tunnel: w98 -> [w122]
            tunnel: w96 -> [w118] mode=indexing
            shift-right: [w127] -> w102
            shift-left: w100 -> [w126]
            shift-right: [w128] -> w103
            shift-left: w99 -> [w125]
            tunnel: w95 -> [w117]
            tunnel: w94 -> [w119]
            tunnel: w90 -> [w114]
            tunnel: w93 -> [w123]
            tunnel: w89 -> [w116]
            tunnel: w92 -> [w115]
            tunnel: w91 -> [w121]
            tunnel: w88 -> [w112]
            tunnel: [w111] -> w86
            tunnel: w84 -> [w110]
            tunnel: w83 -> [w107]
            tunnel: w82 -> [w106]
            tunnel: w81 -> [w105]
            tunnel: [w104] -> w80
            tunnel: w79 -> [_]
            n27 = Bundle By Name(cluster=T6 {"Inspection mode"=FALSE, "Overlay coordinates"=[], "Config coordinates"=[]} ("Fixed FOV parameters"), "Inspection mode"=w107, "Overlay coordinates"=w106, "Config coordinates"=w105) -> (w108:T6)
            n28 = Bundle By Name(cluster=T7 {"Text factor"=0, "Xoffset"=0, "Arc size"=0.0, "Result"=0.0, "Line width"=0, "Measurment Name"="", "Angle"={"Point 1"={"X"=0.0, "Y"=0.0}, "Point 2"={"X"=0.0, "Y"=0.0}, "vertex"={"X"=0.0, "Y"=0.0}, "Point 1a"={"X"=0.0, "Y"=0.0}, "Point 2a"={"X"=0.0, "Y"=0.0}, "line1Point1"={"X"=0.0, "Y"=0.0}, "line1Point2"={"X"=0.0, "Y"=0.0}, "line2Point1"={"X"=0.0, "Y"=0.0}, "line2Point2"={"X"=0.0, "Y"=0.0}, "Angle type"="theta"}, "Maintain Width?"=FALSE, "Size factor"=0, "Colour"=0, "Mouse release point"={"X"=0.0, "Y"=0.0}, "Small FOV?"=FALSE, "Fixed FOV parameters"={"Inspection mode"=FALSE, "Overlay coordinates"=[], "Config coordinates"=[]}} ("Overlay details in"), "Text factor"=w123, "Xoffset"=w122, "Arc size"=w121, "Result"=w120, "Measurment Name"=w119, "Angle"=w118, "Colour"=w117, "Size factor"=w116, "Maintain Width?"=w115, "Line width"=w114, "Mouse release point"=w112, "Small FOV?"=w110, "Fixed FOV parameters"=w108) -> (w113:T7)
            n29 = call "Angle overlay.vi"("error in (no error)"=w126, "Overlay details in"=w113, "Image in"=w125) -> ("error out"=w127:errorcluster, "Overlay Coordinates out"=w104:cluster{"X":sgl, "Y":sgl}[], "Text origin"=w111:cluster{"X":sgl, "Y":sgl}, "Image out"=w128:T5)  [unwired: 5 in]
          }
          n30 = Bundle By Name(cluster=w87, "Text Origin"=w86, "Overlay Coordinates"=w80) -> (w85:T2)
        }
        frame "CircleDia", "CircleRadius" {
          n31 = Unbundle By Name(w148) -> ("Circle"=w147:T19)
          n32 = for {
            tunnel: w150 -> [w176] mode=indexing
            tunnel: w149 -> [w174]
            tunnel: w147 -> [w162] mode=indexing
            shift-right: [w181] -> w152
            shift-left: w143 -> [w170]
            shift-right: [w180] -> w151
            shift-left: w144 -> [w179]
            tunnel: w146 -> [w177]
            tunnel: w145 -> [w158]
            tunnel: w142 -> [w163]
            tunnel: w141 -> [w173]
            tunnel: w140 -> [w159]
            tunnel: w134 -> [w172]
            tunnel: w139 -> [w175]
            tunnel: w138 -> [w161]
            tunnel: [w160] -> w137
            tunnel: w133 -> [w157]
            tunnel: [w156] -> w132
            tunnel: w131 -> [w155]
            tunnel: w130 -> [w154]
            tunnel: w129 -> [w153]
            n33 = call "Calculate angle of intersection(Circle).vi"("error in (no error)"=w170, "Circle"=w162, "Pixel density"=w163, "Input point"=w161) -> ("error out"=w169:errorcluster, "Sleeping line start point"=w165:cluster{"X":sgl, "Y":sgl}, "slanting line start poing"=w166:cluster{"X":sgl, "Y":sgl}, "Angle"=w168:sgl)  [unwired: 4 in]
            n34 = Bundle By Name(cluster=T9 {"slanting line start poing"={"X"=0.0, "Y"=0.0}, "Sleeping line start point"={"X"=0.0, "Y"=0.0}} ("Input points"), "slanting line start poing"=w166, "Sleeping line start point"=w165) -> (w164:T9)
            n35 = Bundle By Name(cluster=T8 {"Overlay shift"=0.0, "Xoffset"=0, "Arc size"=0.0, "Measurement type"="", "Result"=0.0, "Text size factor"=0, "Measurment Name"="", "Colour"=0, "Pixel density"=0.0, "Circle"={"Point 1"={"X"=0.0, "Y"=0.0}, "Point 2"={"X"=0.0, "Y"=0.0}, "Center (Pixels)"={"X"=0.0, "Y"=0.0}, "Radius (Pixels)"=0.0}, "Line width"=0, "Input points"={"slanting line start poing"={"X"=0.0, "Y"=0.0}, "Sleeping line start point"={"X"=0.0, "Y"=0.0}}, "Mouse coordinates"={"X"=0.0, "Y"=0.0}, "Size factor"=0.0, "Inspect Overlay Coordinates"=[], "Config Overlay Coordinates"=[]} ("Cluster in"), "Text size factor"=w173, "Xoffset"=w174, "Arc size"=w175, "Measurement type"=w159, "Result"=w176, "Measurment Name"=w158, "Circle"=w162, "Colour"=w177, "Pixel density"=w163, "Line width"=w172, "Overlay shift"=w168, "Input points"=w164, "Mouse coordinates"=w161, "Size factor"=w157, "Inspect Overlay Coordinates"=w155, "Config Overlay Coordinates"=w153) -> (w171:T8)
            n36 = call "Circle dia adjust.vi"("error in (no error)"=w169, "Inspection \nmode?"=w154, "Cluster in"=w171, "Image in"=w179) -> ("error out"=w181:errorcluster, "Overlay Coordinates"=w156:cluster{"X":sgl, "Y":sgl}[], "Text origin"=w160:cluster{"X":sgl, "Y":sgl}, "Image out"=w180:T5)  [unwired: 4 in]
          }
          n37 = Bundle By Name(cluster=w135, "Text Origin"=w137, "Overlay Coordinates"=w132) -> (w136:T2)
        }
        frame "CircleDatum" {
          n38 = Unbundle By Name(w201) -> ("Circle"=w196:T19)
          n39 = for {
            tunnel: w202 -> [w229]
            tunnel: w196 -> [w220] mode=indexing
            shift-right: [w232] -> w204
            shift-left: w195 -> [w226]
            shift-right: [w231] -> w203
            shift-left: w197 -> [w222]
            tunnel: w200 -> [w227]
            tunnel: w199 -> [w215]
            tunnel: w198 -> [w230]
            tunnel: w194 -> [w221]
            tunnel: w193 -> [w228]
            tunnel: w192 -> [w214]
            tunnel: [w216] -> _
            tunnel: w188 -> [w213]
            tunnel: w187 -> [w212]
            tunnel: w186 -> [w210]
            tunnel: w185 -> [w209]
            tunnel: w184 -> [w208]
            tunnel: [w206] -> w183
            tunnel: w182 -> [w205]
            n40 = call "Calculate angle of intersection(Circle).vi"("error in (no error)"=w226, "Circle"=w220, "Pixel density"=w221, "Input point"=w214) -> ("error out"=w225:errorcluster, "Sleeping line start point"=w217:cluster{"X":sgl, "Y":sgl}, "slanting line start poing"=w218:cluster{"X":sgl, "Y":sgl}, "Angle"=w219:sgl)  [unwired: 4 in]
            n41 = Bundle By Name(cluster=T10 {"Overlay coordinates"=[], "Config coordinates"=[], "Inspection mode?"=FALSE} ("Fixed overlay details"), "Overlay coordinates"=w210, "Config coordinates"=w209, "Inspection mode?"=w208) -> (w207:T10)
            n42 = Bundle By Name(cluster=T11 {"Angle"=315.0, "Reference"="A", "Xoffset"=0, "Arc size"=6.0, "Measurment Name"="CircleDatum", "Pixel density"=3.8423564471879286, "Circle"={"Point 1"={"X"=6458.0, "Y"=4654.0}, "Point 2"={"X"=6458.0, "Y"=4654.0}, "Center (Pixels)"={"X"=5133.0, "Y"=4717.0}, "Radius (Pixels)"=1400.0}, "Color"=16748288, "Slanting line start"={"X"=0.0, "Y"=0.0}, "Sleeping line start"={"X"=0.0, "Y"=0.0}, "Mouse release"={"X"=0.0, "Y"=0.0}, "Line width"=0, "Small FOV?"=FALSE, "Fixed overlay details"={"Overlay coordinates"=[], "Config coordinates"=[], "Inspection mode?"=TRUE}, "PM angle"=0.0} ("Details in"), "Mouse release"=w214, "Angle"=w219, "Reference"=w230, "Xoffset"=w229, "Arc size"=w228, "Measurment Name"=w215, "Pixel density"=w221, "Circle"=w220, "Color"=w227, "Slanting line start"=w218, "Sleeping line start"=w217, "Line width"=w213, "Small FOV?"=w212, "Fixed overlay details"=w207, "PM angle"=w205) -> (w223:T11)
            n43 = call "Datum draw.vi"("error in (no error)"=w225, "Details in"=w223, "Image in"=w222) -> ("error out"=w232:errorcluster, "Overlay coordinates out"=w206:cluster{"X":dbl, "Y":dbl}[], "Text origin"=w216:cluster{"X":sgl, "Y":sgl}, "Image out"=w231:T5)  [unwired: 5 in]
          }
          n44 = Bundle By Name(cluster=w191, "Text Origin"=cluster{"X":dbl, "Y":dbl} {"X"=nan, "Y"=nan}, "Overlay Coordinates"=w183) -> (w190:T2)
        }
        frame "Circularity", "Concentricity", "Parallelism", "Perpendicularity", "Straightness", "Symmetricity" {
          n45 = case shown="\"Others\", Default" w252 {
            tunnel: w255 -> [w261 w268]
            tunnel: [w259 w267] -> w251
            frame "Others", Default {
              n46 = Unbundle By Name(w261) -> ("Line"=w260:T20)
              n47 = for {
                tunnel: w260 -> [w265] mode=indexing
                tunnel: [w262] -> w259 mode=indexing
                n48 = Unbundle By Name(w265) -> ("Point 1"=w264:cluster{"X":sgl, "Y":sgl}, "Point 2"=w263:cluster{"X":sgl, "Y":sgl})
                n49 = Bundle By Name(cluster=T12 {"Point 1"={"X"=0.0, "Y"=0.0}, "Point 2"={"X"=0.0, "Y"=0.0}, "Center (Pixels)"={"X"=0.0, "Y"=0.0}, "Radius (Pixels)"=0.0} ("Circle"), "Point 1"=w264, "Point 2"=w263) -> (w262:T12)
              }
            }
            frame "Circularity", "Concentricity", "Datum" {
              n50 = Unbundle By Name(w268) -> ("Circle"=w267:T19)
            }
          }
          n51 = for {
            tunnel: w247 -> [w289] mode=indexing
            tunnel: w256 -> [w290]
            tunnel: w251 -> [w284] mode=indexing
            shift-right: [w296] -> w258
            shift-left: w248 -> [w280]
            shift-right: [w295] -> w257
            shift-left: w249 -> [w294]
            tunnel: w254 -> [w287]
            tunnel: 315.0 -> [w283]
            tunnel: w253 -> [w288]
            tunnel: w252 -> [w281]
            tunnel: w250 -> [w292]
            tunnel: w246 -> [w277]
            tunnel: w245 -> [w291]
            tunnel: w244 -> [_]
            tunnel: w243 -> [w286]
            tunnel: w241 -> [w278]
            tunnel: [w274] -> w239
            tunnel: [w273] -> w237
            tunnel: w236 -> [w272]
            tunnel: w235 -> [w271]
            tunnel: w234 -> [w270]
            tunnel: w233 -> [w269]
            n52 = case shown="\"Others\", Default" w281 {
              tunnel: w284 -> [w298 w309]
              tunnel: w283 -> [_ w308]
              tunnel: [w303 w307] -> w282
              tunnel: w278 -> [_ w306]
              tunnel: w280 -> [w297 w305]
              tunnel: [w304 w305] -> w279
              tunnel: w278 -> [w302 _]
              tunnel: w277 -> [w301 _]
              tunnel: [w300 _] -> w276
              tunnel: [w299 _] -> w275
              frame "Circularity", "Concentricity" {
                n53 = call "Calculate angle of intersection(Circle).vi"("error in (no error)"=w297, "Circle"=w298, "Pixel density"=w301, "Input point"=w302) -> ("error out"=w304:errorcluster, "Sleeping line start point"=w299:cluster{"X":sgl, "Y":sgl}, "slanting line start poing"=w300:cluster{"X":sgl, "Y":sgl}, "Angle"=w303:sgl)  [unwired: 4 in]
              }
              frame "Others", Default {
                n54 = call "Calculate angle.vi"("Mouse release coordinates"=w306, "Circle"=w309, "Angle (in degrees)"=w308) -> ("Angle"=w307:dbl)  [unwired: 8 in]
              }
            }
            n55 = Bundle By Name(cluster=T13 {"Overlay shift"=0.0, "Reference"="", "Arc size"=0.0, "Measurement type"="", "Xoffset"=0, "Result"=0.0, "Measurment Name"="", "Color"=0, "Points"={"Point 1"={"X"=0.0, "Y"=0.0}, "Point 2"={"X"=0.0, "Y"=0.0}, "Center (Pixels)"={"X"=0.0, "Y"=0.0}, "Radius (Pixels)"=0.0}, "Pixel density"=0.0, "Line width"=0, "Mouse release point"={"X"=0.0, "Y"=0.0}, "Slanting start point"={"X"=0.0, "Y"=0.0}, "Sleeping start point"={"X"=0.0, "Y"=0.0}, "Small FOV?"=FALSE, "Fixed overlays"={"Overlay coordinates"=[], "Config coordinates"=[], "Inspection mode"=FALSE}, "Angle of rotation"=0.0} ("Overlay details in"), "Reference"=w292, "Overlay shift"=w282, "Arc size"=w291, "Measurement type"=w281, "Xoffset"=w290, "Result"=w289, "Measurment Name"=w288, "Color"=w287, "Points"=w284, "Pixel density"=w277, "Line width"=w286, "Mouse release point"=w278, "Slanting start point"=w276, "Sleeping start point"=w275, "Fixed overlays.Overlay coordinates"=w272, "Fixed overlays.Config coordinates"=w271, "Fixed overlays.Inspection mode"=w270, "Angle of rotation"=w269) -> (w285:T13)
            n56 = call "Overlay GD & T.vi"("error in (no error)"=w279, "Overlay details in"=w285, "Image in"=w294) -> ("error out"=w296:errorcluster, "Overlay coordinates"=w273:cluster{"X":dbl, "Y":dbl}[], "Text origin"=w274:cluster{"X":dbl, "Y":dbl}, "Image out"=w295:T5)  [unwired: 5 in]
          }
          n57 = Bundle By Name(cluster=w240, "Text Origin"=w239, "Overlay Coordinates"=w237) -> (w238:T2)
        }
        frame "LineSeg" {
          w320 = 0.0 ("Overlay shift1")
          w326 = T21 {"Arrow head diverge angle"=0.0, "Arrow height"=0.0, "Line width"=0, "Maintain Width?"=FALSE, "Text factor"=0}  # Calculated inputs (line)
          w328 = T22 {"Measurement name"="A", "Line"={"Point 1"={"X"=0.0, "Y"=0.0}, "Point 2"={"X"=0.0, "Y"=0.0}}, "Result"=0.0, "Overlay shift1"=0.0, "Overlay shift2"=0.0, "Allign Text With Overlay"=FALSE, "Overlay text position"="A", "Color"=0, "Xoffset"=0, "Size factor"=0.0, "Inspection mode?"=FALSE, "Configuration overlay coordinates"=[]}  # User inputs (line)
          n58 = Unbundle By Name(w344) -> ("Points"=w343:cluster{"Points":cluster{"X":sgl, "Y":sgl}[]})
          n59 = Index Array(array=w341) -> (element=w340:sgl)  [unwired: 1 in]
          n60 = Unbundle By Name(w343) -> ("Points"=w319:cluster{"X":sgl, "Y":sgl}[])
          n61 = call "Overlay adjust (line).vi"("Image in"=w349, "Enable overlay?"=FALSE, "Measurement Name"=w331, "Configured coordinates"=w316, "Mouse release point"=w332, "Line width"=w318, "Points array"=w319, "error in (no error)"=w346, "Color"=w342, "Inspection mode"=w315, "Overlay coordinates"=w314) -> ("Image Out"=w323:T5, "Transformed line"=w322:T23, "Overlay Coordinates"=w312:cluster{"X":sgl, "Y":sgl}[], "error out"=w324:errorcluster)  [unwired: 1 out]
          n62 = Bundle By Name(cluster=w328, "Overlay text position"=w336, "Allign Text With Overlay"=w335, "Overlay shift1"=w320, "Overlay shift2"=w320, "Xoffset"=w345, "Result"=w340, "Measurement name"=w331, "Color"=w342, "Line"=w322, "Size factor"=w318, "Inspection mode?"=w315, "Configuration overlay coordinates"=w316) -> (w327:T22)
          n63 = Bundle By Name(cluster=w326, "Text factor"=w339, "Arrow height"=w337, "Arrow head diverge angle"=w338, "Maintain Width?"=w334, "Line width"=w333) -> (w325:T21)
          n64 = call "Overlay line segment.vi"("Overlay Coordinates"=w314, "error in (no error)"=w324, "Calculated inputs (line)"=w325, "User inputs (line)"=w327, "Image in"=w323) -> ("error out"=w347:errorcluster, "Overlay coordinates"=w311:cluster{"X":sgl, "Y":sgl}[], "Text origin"=w317:cluster{"X":sgl, "Y":sgl}, "Image out"=w348:T5)  [unwired: 2 in, 1 out]
          n65 = Insert Into Array(array=cluster{"X":sgl, "Y":sgl}[] [], new element #1=w312, new element #2=w311) -> (w310:cluster{"X":sgl, "Y":sgl}[])  [unwired: 1 in]
          n66 = Bundle By Name(cluster=w329, "Text Origin"=w317, "Overlay Coordinates"=w310) -> (w330:T2)
        }
        frame "Coordinate system" {
          n67 = Unbundle By Name(w359) -> ("Coordinate System"=w358:T24)
          n68 = Bundle By Name(cluster=T14 {"Arrow height"=0.0, "Measurment Name"="", "Coordinate System"={"Origin"={"X"=0.0, "Y"=0.0}, "Angle (deg)"=0.0, "Axis Reference"=0}, "Color"=0, "Width"=0, "Arrow angle in"=0.0, "SmallFOV?"=FALSE} ("Details in"), "Arrow height"=w361, "Measurment Name"=w360, "Coordinate System"=w358, "Color"=w357, "Width"=w356, "Arrow angle in"=w355, "SmallFOV?"=w350) -> (w354:T14)
          n69 = call "Draw coordinate reference.vi"("error in (no error)"=w353, "Details in"=w354, "Image in"=w362) -> ("error out"=w363:errorcluster, "Image out"=w364:T5)  [unwired: 7 in]
        }
        frame "LineDatum" {
          n70 = Unbundle By Name(w384) -> ("Line"=w383:T20)
          n71 = for {
            tunnel: w383 -> [w407] mode=indexing
            tunnel: w382 -> [w415]
            shift-right: [w421] -> w378
            shift-left: w379 -> [w410]
            shift-right: [w419] -> w380
            shift-left: w381 -> [w434]
            tunnel: w376 -> [w424]
            tunnel: w377 -> [w423]
            tunnel: w375 -> [w418]
            tunnel: w374 -> [w406]
            tunnel: [w402] -> _
            tunnel: w370 -> [w401]
            tunnel: w369 -> [w394]
            tunnel: w368 -> [w387]
            tunnel: w367 -> [w396]
            tunnel: [w397] -> w366
            tunnel: w365 -> [w386]
            w411 = u32 2  # Width
            w412 = TRUE  # Maintain Width?
            w413 = u16 30  # Arrow height (in pixels)
            w414 = u16 40  # half Datum arrow width( in pixels)
            n72 = Unbundle By Name(w407) -> ("Point 1"=w417:cluster{"X":sgl, "Y":sgl}, "Point 2"=w416:cluster{"X":sgl, "Y":sgl})
            n73 = Unbundle By Name(w417) -> ("Y"=w427:sgl, "X"=w429:sgl)
            n74 = Unbundle By Name(w416) -> ("Y"=w428:sgl, "X"=w430:sgl)
            n75 = Add(x=w417, y=w416) -> (x+y=w425:cluster{"X":sgl, "Y":sgl})
            n76 = Subtract(x=w427, y=w428) -> (x-y=w433:sgl)
            n77 = Bundle By Name(cluster=T10 {"Overlay coordinates"=[], "Config coordinates"=[], "Inspection mode?"=TRUE} ("Fixed overlay details"), "Overlay coordinates"=w394, "Config coordinates"=w387, "Inspection mode?"=w396) -> (w399:T10)
            n78 = Subtract(x=w429, y=w430) -> (x-y=w431:sgl)
            n79 = Divide(x=w425, y=cluster{"X":sgl, "Y":sgl} {"X"=2.0, "Y"=2.0}) -> (x/y=w408:cluster{"X":sgl, "Y":sgl})
            n80 = Divide(x=w433, y=w431) -> (x/y=w432:sgl)
            n81 = Inverse Tangent(1:w432) -> (0:w403:sgl)
            n82 = call "Calculate sleeping line length_datumLine.vi"("Datum angle"=w403, "error in (no error)"=w410, "Datum origin"=w408, "Line"=w407, "Mouse release \npoint"=w406) -> ("error out"=w409:errorcluster, "Angle offset"=w404:dbl, "Slanting line\nlength"=w405:sgl)  [unwired: 4 in]
            n83 = Index Array(array=w394, index #1=13 ("index")) -> (element #1=w392:cluster{"X":sgl, "Y":sgl}, element #2=w391:cluster{"X":sgl, "Y":sgl})  [unwired: 1 in]
            n84 = Insert Into Array(array=cluster{"X":sgl, "Y":sgl}[] [], new element #1=w392, new element #2=w391) -> (w389:cluster{"X":sgl, "Y":sgl}[])  [unwired: 1 in]
            n85 = call "Line Datum.vi"("Image in"=w434, "Small FOV?"=w401, "Angle of rotation"=w386, "half Datum arrow width( in pixels)"=w414, "Arrow height (in pixels)"=w413, "Datum origin"=w408, "Start index"=6, "error in (no error)"=w409, "Color"=w415, "Datum line angle"=w404, "Angular line length(in pixels)"=w405, "pixel factor"=w424, "Reference string"=w423, "Measurement name"=w418, "Fixed overlay details"=w399) -> ("Image out"=w420:T5, "Text origin out"=w402:cluster{"X":sgl, "Y":sgl}, "Overlay coordinates out"=w398:cluster{"X":dbl, "Y":dbl}[], "error out"=w422:errorcluster)  [unwired: 9 in]
            n86 = Build Array(w417, w416) -> (w395:cluster{"X":sgl, "Y":sgl}[])
            n87 = Select(t=w389, s=w396, f=w395) -> (s? t:f=w388:cluster{"X":sgl, "Y":sgl}[])
            n88 = case shown="False" w396 {
              tunnel: w398 -> [w438 _]
              tunnel: w395 -> [w436 _]
              tunnel: [w435 w439] -> w397
              tunnel: w387 -> [_ w439]
              frame False {
                n89 = Insert Into Array(array=cluster{"X":dbl, "Y":dbl}[] [], new element #1=w438, new element #2=w436) -> (w435:cluster{"X":dbl, "Y":dbl}[])  [unwired: 1 in]
              }
              frame True {
              }
            }
            n90 = call "IMAQ Overlay Multiple Lines 2"("Image"=w420, "Group"=w418, "Line End Points"=w388, "Color"=w415, "error in (no error)"=w422, "Maintain Width?"=w412, "Width"=w411) -> ("Image Out"=w419:T5, "error out"=w421:errorcluster)  [unwired: 7 in]
          }
          n91 = Bundle By Name(cluster=w373, "Overlay Coordinates"=w366, "Text Origin"=cluster{"X":dbl, "Y":dbl} {"X"=nan, "Y"=nan}) -> (w372:T2)
        }
        frame "Point" {
          n92 = Unbundle By Name(w449) -> ("Points.Points"=w447:cluster{"X":sgl, "Y":sgl}[])
          n93 = call "Overlay Points with User Specified Size.vi"("Color"=w443, "Group"=w442, "error in"=w448, "Point Diameter (5)"=w441, "Points"=w447, "Image In"=w446) -> ("error out"=w445:errorcluster, "Image Out"=w444:T5)  [unwired: 4 in]
        }
        frame "Line" {
          # "line multiplication factor"
          n94 = Unbundle By Name(w455) -> ("Line"=w454:T20)
          n95 = for {
            tunnel: w452 -> [w460]
            tunnel: w454 -> [w472] mode=indexing
            shift-right: [w470] -> w456
            shift-left: w459 -> [w471]
            shift-right: [w463] -> w457
            shift-left: w458 -> [w468]
            tunnel: w453 -> [w469]
            tunnel: w451 -> [w461]
            n96 = Unbundle By Name(w472) -> ("Point 1"=w466:cluster{"X":sgl, "Y":sgl}, "Point 2"=w465:cluster{"X":sgl, "Y":sgl})
            n97 = Insert Into Array(array=cluster{"X":dbl, "Y":dbl}[] [] ("Line End Points"), new element #1=w466, new element #2=w465) -> (w464:cluster{"X":dbl, "Y":dbl}[])  [unwired: 1 in]
            n98 = call "IMAQ Overlay Multiple Lines 2"("Image"=w468, "Group"=w469, "Line End Points"=w464, "Color"=w460, "error in (no error)"=w471, "Maintain Width?"=TRUE, "Width"=w461) -> ("Image Out"=w463:T5, "error out"=w470:errorcluster)  [unwired: 7 in]
          }
        }
        frame "Circle" {
          n99 = Unbundle By Name(w485) -> ("Circle"=w484:T19)
          n100 = for {
            tunnel: w484 -> [w489] mode=indexing
            shift-right: [w497] -> w482
            shift-left: w483 -> [w498]
            tunnel: w481 -> [w493]
            tunnel: w480 -> [w487]
            tunnel: w479 -> [w488]
            shift-right: [w496] -> w478
            shift-left: w477 -> [w495]
            tunnel: w476 -> [w490]
            tunnel: w475 -> [w492]
            tunnel: w474 -> [w491]
            n101 = Bundle By Name(cluster=T15 {"Xoffset"=0, "Point size"=0.0, "Arc size"=0.0, "Measurment Name"="", "Circle"={"Point 1"={"X"=0.0, "Y"=0.0}, "Point 2"={"X"=0.0, "Y"=0.0}, "Center (Pixels)"={"X"=0.0, "Y"=0.0}, "Radius (Pixels)"=0.0}, "Color"=0, "Line width"=0} ("Detail in"), "Xoffset"=w493, "Point size"=w492, "Arc size"=w491, "Measurment Name"=w490, "Circle"=w489, "Color"=w488, "Line width"=w487) -> (w486:T15)
            n102 = call "Draw circle.vi"("error in (no error)"=w498, "Detail in"=w486, "Image in"=w495) -> ("error out"=w497:errorcluster, "Image out"=w496:T5)  [unwired: 7 in]
          }
        }
      }
    }
    frame Error {
    }
  }
  "Image Out" <- w10
  "Overlay output" <- w2
  n103 = call <vilib>:"Clear Errors.vi"("error in (no error)"=w5) -> ("error out"=→"error out":errorcluster)  [unwired: 5 in, 1 out]
